vi "FPGAAddon.SpecialityOutputs.Generate.vi"(8 "error in (no error)":errorcluster, 11 "Parameters":T1) -> (0 "error out":errorcluster, 3 "Output.Ref":refnum<vi>)   [LabVIEW 2015]
uses:
  FPGAAddon.SpecialityOutputs.Generate.Parameters.ctl
  <vilib>/Utility/miscctls.llb/LVPointTypeDef.ctl
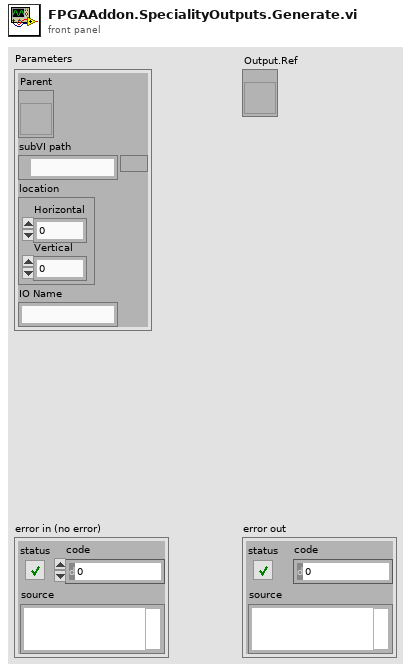
[diagram p1: front panel]
types:
  T1 = typedef "FPGAAddon.SpecialityOutputs.Generate.Parameters.ctl" = cluster{"Parent":refnum<vi>, "subVI path":path, "location":T2, "IO Name":string}
  T2 = typedef "LVPointTypeDef.ctl" = cluster{"Horizontal":i16, "Vertical":i16}
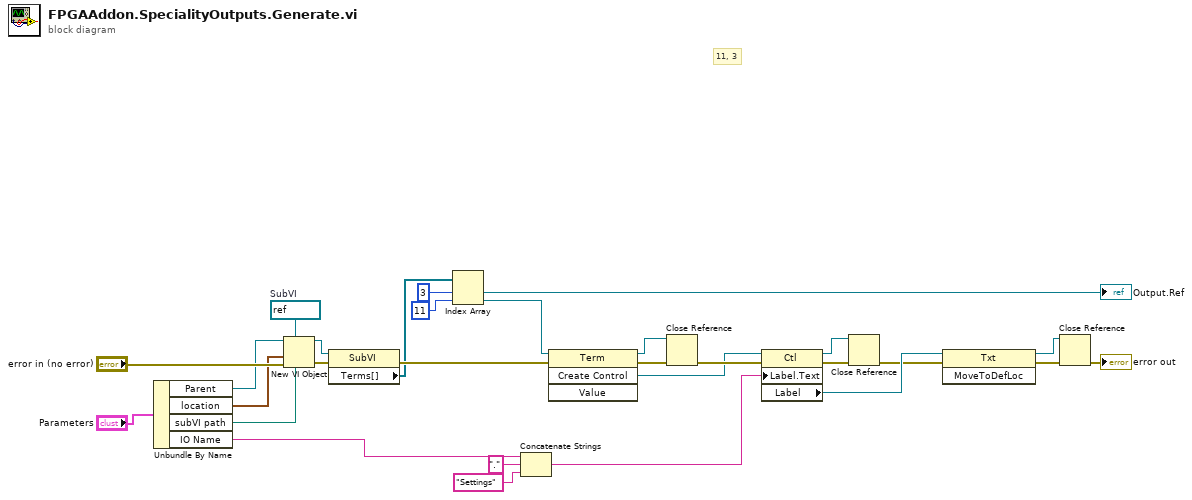
[diagram p0: block diagram]
diagram:
  w15 = refnum<vi> refnum  # SubVI
  # "11, 3"
  n1 = Unbundle By Name("Parameters") -> ("Parent"=w13:refnum<vi>, "location"=w12:T2, "subVI path"=w11:path, "IO Name"=w10:string)
  n2 = New VI Object(vi object class=w15, owner refnum=w13, position/next to=w12, 6:w11, 8:"error in (no error)") -> (object refnum=w20:refnum<vi>, 0:w21:errorcluster)  [unwired: 3 in]
  n3 = property class="SubVI"(reference=w20, error in=w21) -> (error out=w22:errorcluster, "Terms[]"=w17:refnum<vi>[])  [unwired: 1 out]
  n4 = Index Array(array=w17, index #1=3 ("index"), index #2=11 ("index")) -> (element #1=→"Output.Ref":refnum<vi>, element #2=w2:refnum<vi>)
  n5 = Concatenate Strings(w10, "." ("string"), "Settings" ("string")) -> (w23:string)
  n6 = invoke class="Term" method="Create Control"(reference=w2, error in=w22) -> (reference out=w27:refnum<vi>, error out=w26:errorcluster, "Create Control"=w9:refnum<vi>)  [unwired: 2 in, 1 out]
  n7 = Close Reference(reference=w27, error in (no error)=w26) -> (error out=w28:errorcluster)
  n8 = property class="Ctl"(reference=w9, error in=w28, "Label.Text"=w23) -> (reference out=w8:refnum<vi>, error out=w6:errorcluster, "Label"=w7:refnum<vi>)
  n9 = Close Reference(reference=w8, error in (no error)=w6) -> (error out=w5:errorcluster)
  n10 = invoke class="Txt" method="MoveToDefLoc"(reference=w7, error in=w5) -> (reference out=w3:refnum<vi>, error out=w4:errorcluster)  [unwired: 1 in, 1 out]
  n11 = Close Reference(reference=w3, error in (no error)=w4) -> (error out=→"error out":errorcluster)
